vi "Save VI to File.vi"(8 "错误输入（无错误）":errorcluster, 10 "保存文件的路径":path, 11 "VI Ref":refnum<vi>) -> (0 "错误输出":errorcluster)   [LabVIEW 2012, in "VIRef.lvlib"]
uses:
  VIRef.lvlib
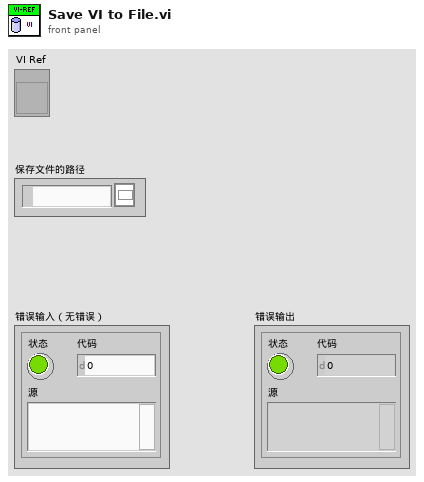
[diagram p1: front panel]
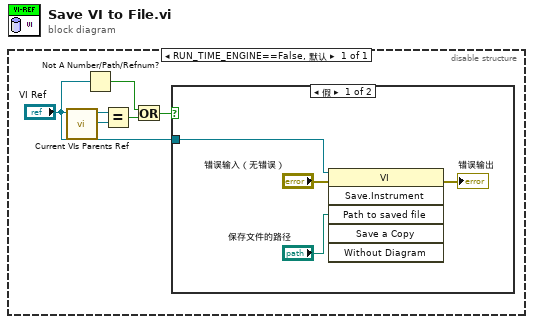
[diagram p0: block diagram]
diagram:
  n1 = disable-structure shown="RUN_TIME_ENGINE==False, 默认" {
    frame condition #0 (active) {
      n2 = call "Current VIs Parents Ref.vi"() -> ("Calling VI's Reference"=w5:refnum<vi>)  [unwired: 2 in]
      n3 = Not A Number/Path/Refnum?(number/path/refnum="VI Ref") -> (NaN/Path/Refnum?=w4:bool)
      n4 = Equal?(x="VI Ref", y=w5) -> (x = y?=w3:bool)
      n5 = Or(x=w4, y=w3) -> (x .or. y?=w2:bool)
      n6 = case shown="假" w2 {
        tunnel: "VI Ref" -> [w6 _]
        frame False {
          n7 = invoke class="VI" method="Save.Instrument"(reference=w6, error in="错误输入（无错误）", "Path to saved file"="保存文件的路径") -> (error out=→"错误输出":errorcluster)  [unwired: 3 in, 5 out]
        }
        frame True {
        }
      }
    }
  }
